vi "SLSC System Property Node.vi"   [LabVIEW 2020]
doc: "A Property Node with the SLSC System class preselected. This can be used to query which devices are available on the system, without initializing a session."
uses:
  <resource>/objmgr/slsc.rc
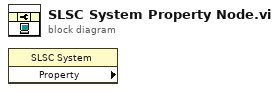
[diagram p0: block diagram]
diagram:
  n1 = property class="SLSC System" props=[]() -> ()  [unwired: 2 in, 3 out]
